vi "APXPressureReaderEPICS.vi"() -> ()   [LabVIEW 2015]
uses:
  <vilib>/Instr/_visa.llb/VISA Configure Serial Port (Instr).vi
  <userlib>/caLab/Private/Get_PV-1D.vi
  <userlib>/caLab/Private/Put_DBL-1D_PV-1D.vi
panel:
  out "VISA resource name out":refnum<visa-resource-name>
  out "APX:Gas":dbl format="%_3f"
  out "APX:Gas2":dbl format="%_3f"
  out "read buffer Main":string
  out "COM MAXGAUGE":refnum<visa-resource-name>
  out "Status":bool
  out "APX:SP_F":bool
  out "APX:SP_E":bool
  out "APX_SP_D":bool
  out "APX:SP_C":bool
  out "APX:SP_B":bool
  out "APX:SP_A":bool
  out "Cycle":i32
  out "Error out":errorcluster
  out "APX:SEN6_VAL":dbl format="%.6f"
  out "APX:SEN5_VAL":dbl format="%#_3e"
  out "APX:SEN4_VAL":dbl format="%#_4g"
  out "APX:SEN3_VAL":dbl format="%#_3g"
  out "APX:SEN2_VAL":dbl format="%#_3g"
  out "APX:SEN1_VAL":dbl format="%.5g"
  out "APX:SEN6_OFF":bool
  out "APX:SEN6_ON":bool
  out "APX:SEN5_OFF":bool
  out "APX:SEN5_ON":bool
  out "APX:SEN4_OFF":bool
  out "APX:SEN4_ON":bool
  out "APX:SEN3_OFF":bool
  out "APX:SEN3_ON":bool
  out "APX:SEN2_OFF":bool
  out "APX:SEN2_ON":bool
  out "APX:SEN1_OFF":bool
  out "APX:SEN1_ON":bool
  in  "STOP":bool
  # "APX:SP_SES100"
  # "APX:HPC100"
  # "APX:HPC"
  # "APX:PREP"
  # "APX:AP1"
  # "APX:AP2"
  # "APX:HPC01"
  # "APX:GAS"
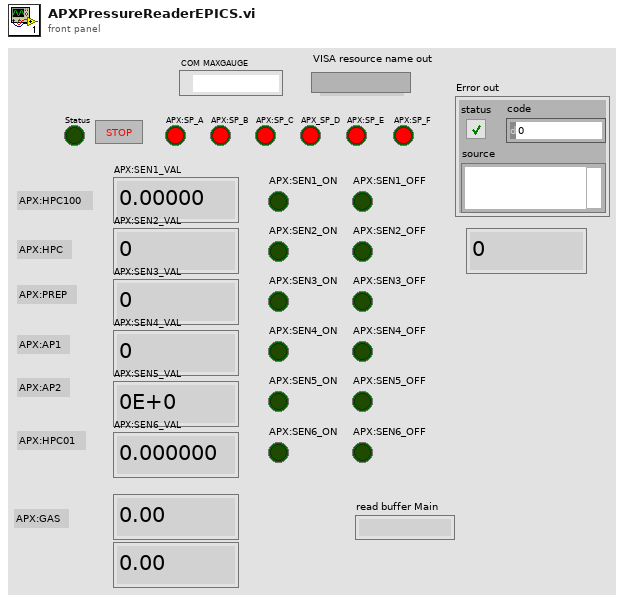
[diagram p1: front panel]
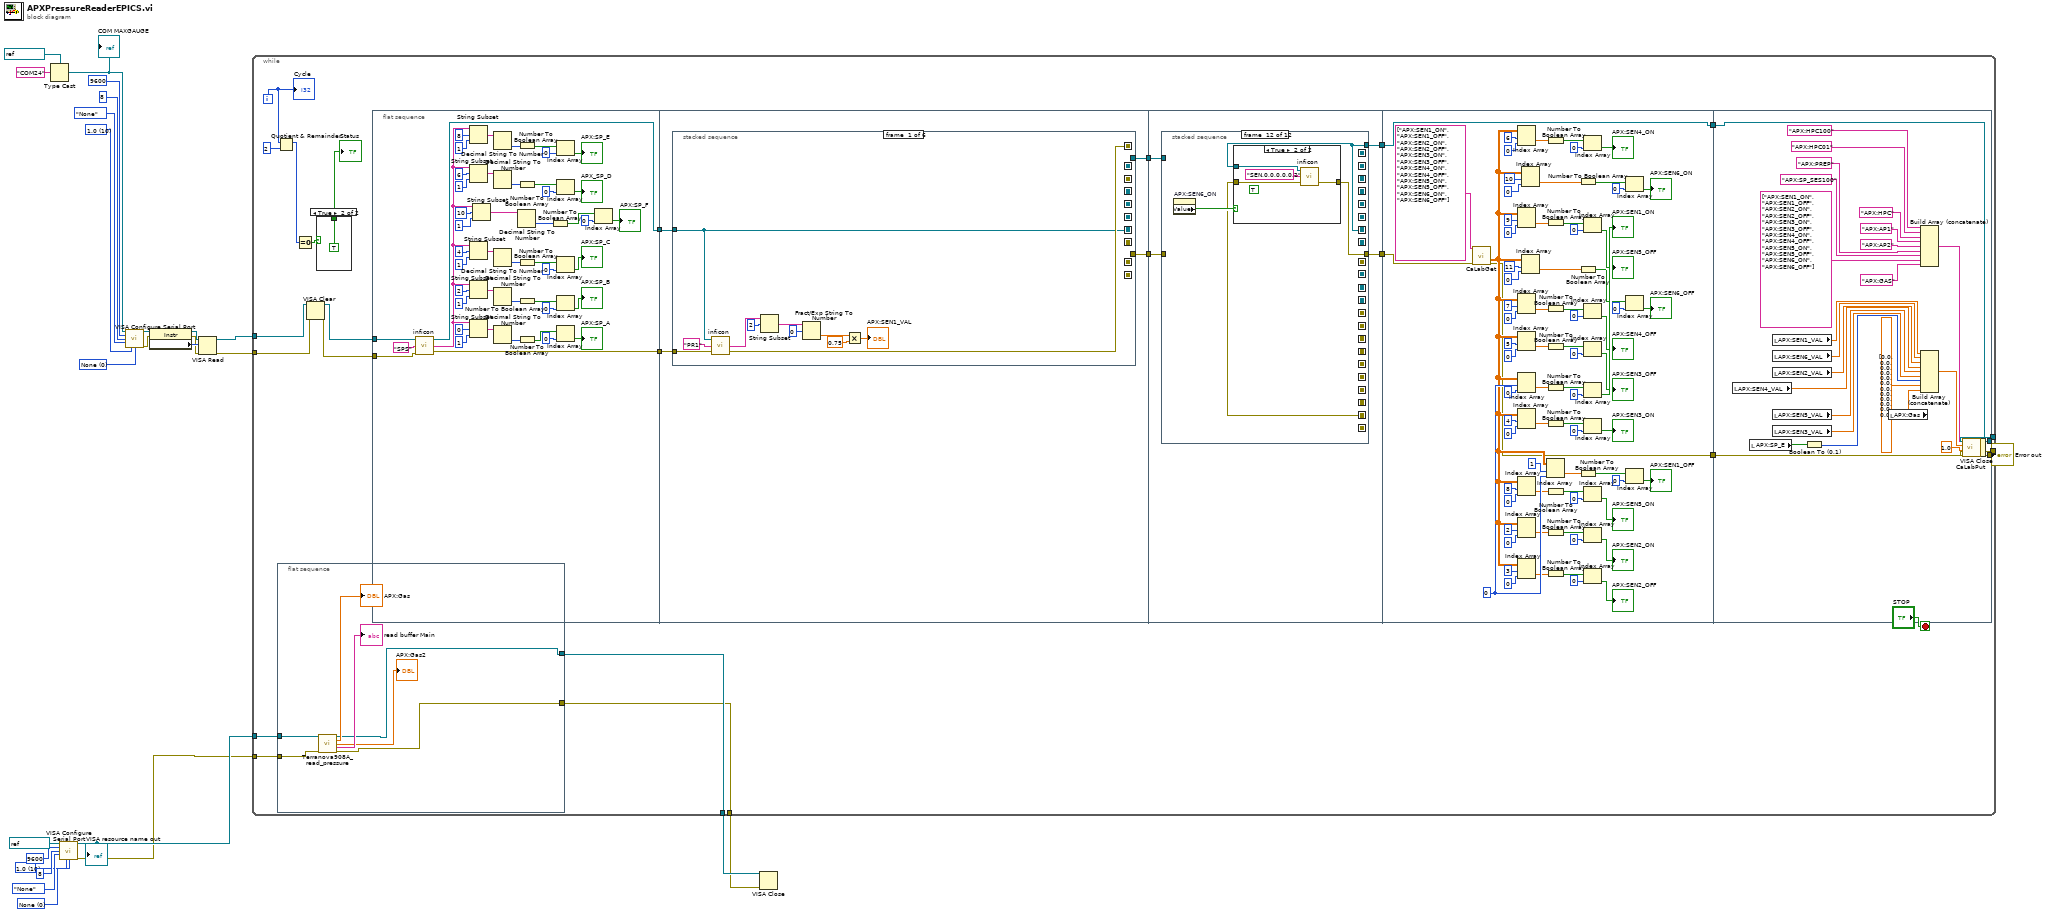
[diagram p0: block diagram]
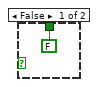
[diagram p2: hidden frame]
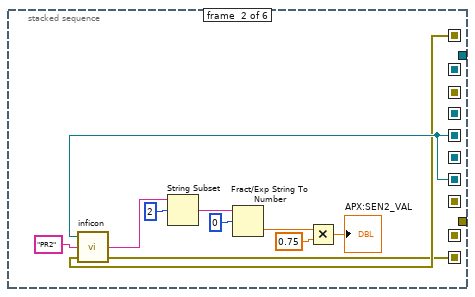
[diagram p3: hidden frame]
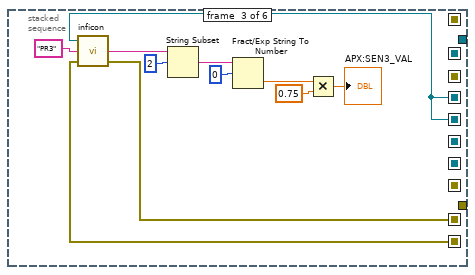
[diagram p4: hidden frame]
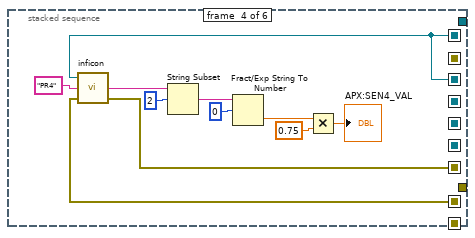
[diagram p5: hidden frame]
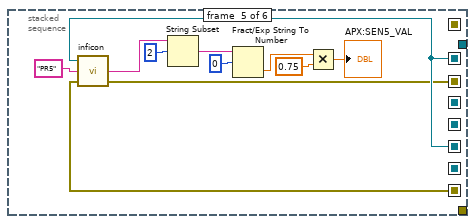
[diagram p6: hidden frame]
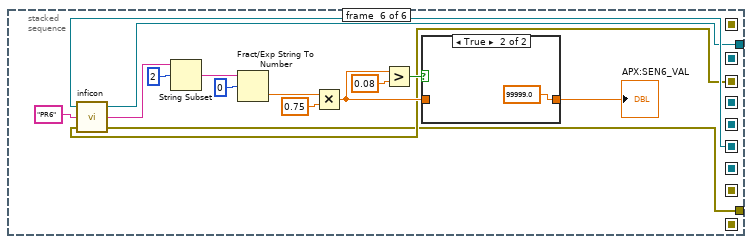
[diagram p7: hidden frame]
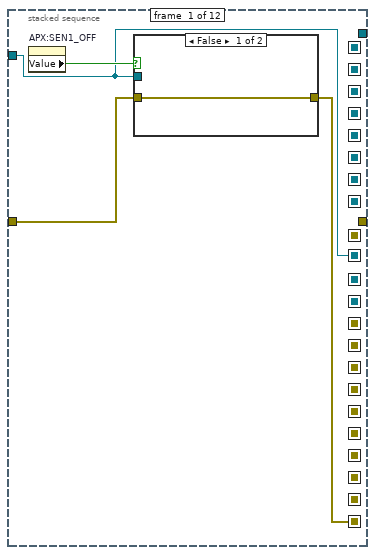
[diagram p9: hidden frame]
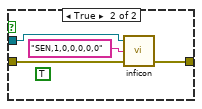
[diagram p10: hidden frame]
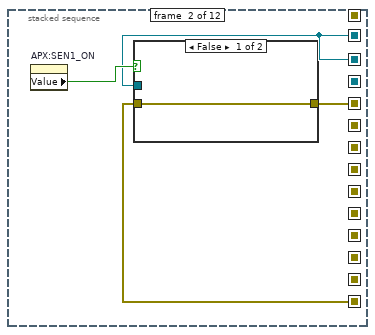
[diagram p11: hidden frame]
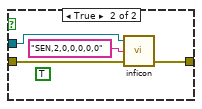
[diagram p12: hidden frame]
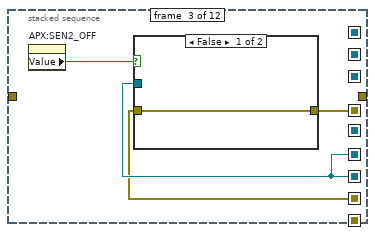
[diagram p13: hidden frame]
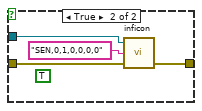
[diagram p14: hidden frame]
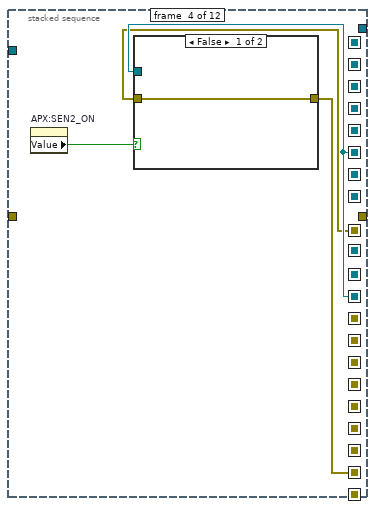
[diagram p15: hidden frame]
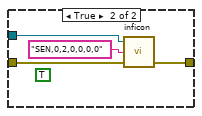
[diagram p16: hidden frame]
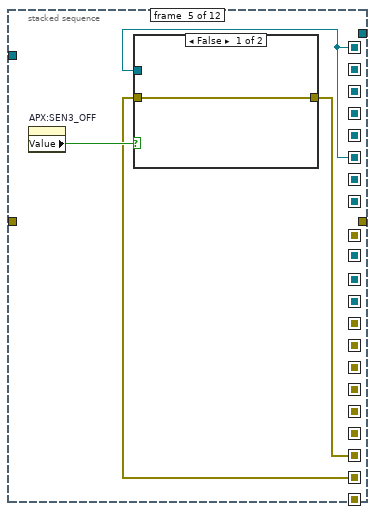
[diagram p17: hidden frame]
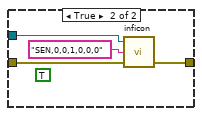
[diagram p18: hidden frame]
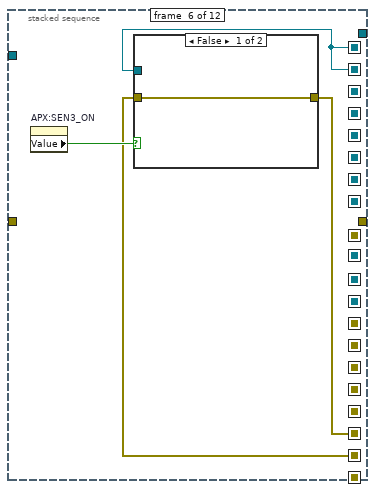
[diagram p19: hidden frame]
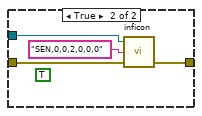
[diagram p20: hidden frame]
diagram:
  w5 = u16 10 items=["1.0"=10, "1.5"=15, "2.0"=20] ("stop bits (10: 1 bit)")
  w6 = u16 0 items=["None", "XON/XOFF", "RTS/CTS", "XON/XOFF & RTS/CTS", "DTR/DSR", "XON/XOFF & DTR/DSR"] ("flow control (0:none)")
  w24 = u16 10 items=["1.0"=10, "1.5"=15, "2.0"=20] ("stop bits (10: 1 bit)")
  w25 = u16 0 items=["None", "XON/XOFF", "RTS/CTS", "XON/XOFF & RTS/CTS", "DTR/DSR", "XON/XOFF & DTR/DSR"] ("flow control (0:none)")
  n1 = Type Cast(type=refnum<visa-resource-name> "COM24" ("VISA resource name"), x="COM24") -> (*(type *) &x=w22:refnum<visa-resource-name>)
  "COM MAXGAUGE" <- w22
  n2 = call-poly "VISA Configure Serial Port"("VISA resource name"=refnum<visa-resource-name> "COM10", "baud rate (9600)"=u32 9600, "data bits (8)"=u16 8, "parity (0:none)"=enum16{"None", "Odd", "Even", "Mark", "Space"}."None", "stop bits (10: 1 bit)"=w5, "flow control (0:none)"=w6) -> ("VISA resource name out"=w2:refnum<visa-resource-name>, "error out"=w1:errorcluster)  [unwired: 8 in]
  "VISA resource name out" <- w2
  n3 = call-poly "VISA Configure Serial Port"("VISA resource name"=w22, "baud rate (9600)"=u32 9600, "data bits (8)"=u16 8, "parity (0:none)"=enum16{"None", "Odd", "Even", "Mark", "Space"}."None", "stop bits (10: 1 bit)"=w24, "flow control (0:none)"=w25) -> ("VISA resource name out"=w19:refnum<visa-resource-name>, "error out"=w11:errorcluster)  [unwired: 8 in]
  n4 = property class="Instr"(reference=w19, error in=w11) -> (reference out=w20:refnum<visa-resource-name>, error out=w12:errorcluster, "Serial Settings:Number of Bytes at Serial Port"=w17:u32)
  n5 = VISA Read(VISA resource name=w20, byte count=w17, error in (no error)=w12) -> (VISA resource name out=w18:refnum<visa-resource-name>, error out=w13:errorcluster)  [unwired: 2 out]
  n6 = while {
    tunnel: [w46] -> w15
    tunnel: w18 -> [w41]
    tunnel: [w49] -> w16
    tunnel: w13 -> [w39]
    tunnel: [w32] -> w4
    tunnel: [w31] -> w3
    tunnel: w2 -> [w30]
    tunnel: w1 -> [w29]
    i -> [w35]
    stop <- "STOP" stop-if-true
    n7 = Quotient & Remainder(x=w35, y=2) -> (x-y*floor(x/y)=w36:i32)  [unwired: 1 out]
    n8 = flat-sequence {
      tunnel: w30 -> [w59]
      tunnel: [w57] -> w31
      tunnel: [w54] -> w32
      tunnel: w29 -> [w53]
      frame #0 {
        n9 = call "Terranova908A_read_pressure.vi"("VISA resource name"=w59, "error in (no error)"=w53) -> ("VISA resource name out"=w54:refnum<visa-resource-name>, "pressure"=→"APX:Gas":dbl, "pressure 2"=→"APX:Gas2":dbl, "read buffer"=→"read buffer Main":string, "error out"=w57:errorcluster)  [unwired: 9 in]
      }
    }
    n10 = Equal To 0?(x=w36) -> (x = 0?=w37:bool)
    n11 = VISA Clear(VISA resource name=w41, error in (no error)=w39) -> (VISA resource name out=w40:refnum<visa-resource-name>, error out=w38:errorcluster)
    n12 = case shown="True" w37 {
      tunnel: [FALSE ("Status") TRUE ("Status")] -> w33
      frame False {
      }
      frame True {
      }
    }
    "Status" <- w33
    n13 = flat-sequence {
      tunnel: w40 -> [w101]
      tunnel: [w100] -> w51
      tunnel: [w63] -> w45
      tunnel: w38 -> [w62]
      tunnel: w51 -> [w112]
      tunnel: [w111] -> w50
      tunnel: w45 -> [w113]
      tunnel: [w110] -> w44
      tunnel: w50 -> [w189]
      tunnel: w44 -> [w188]
      tunnel: [w187] -> w43
      tunnel: [w186] -> w42
      tunnel: [w300] -> w48
      tunnel: [w299] -> w47
      tunnel: w43 -> [w298]
      tunnel: w42 -> [w299]
      tunnel: [w398] -> w49
      tunnel: w48 -> [w376]
      tunnel: w47 -> [w398]
      tunnel: [w377] -> w46
      frame #0 {
        n14 = call "inficon.vi"("error out"=w62, "string to write"="SPS", "VISA resource name"=w101) -> ("error out 2"=w63:errorcluster, "read buffer 2"=w69:string, "VISA resource name 2"=w100:refnum<visa-resource-name>)
        n15 = String Subset(string=w69, offset (0)=8, length (rest)=1 ("length (rest)")) -> (substring=w103:string)
        n16 = String Subset(string=w69, offset (0)=6, length (rest)=1 ("length (rest)")) -> (substring=w88:string)
        n17 = String Subset(string=w69, offset (0)=4, length (rest)=1 ("length (rest)")) -> (substring=w94:string)
        n18 = String Subset(string=w69, offset (0)=2, length (rest)=1 ("length (rest)")) -> (substring=w82:string)
        n19 = String Subset(string=w69, offset (0)=0, length (rest)=1 ("length (rest)")) -> (substring=w76:string)
        n20 = String Subset(string=w69, offset (0)=10, length (rest)=1 ("length (rest)")) -> (substring=w70:string)
        n21 = Decimal String To Number(string=w103) -> (number=w104:i32)  [unwired: 2 in, 1 out]
        n22 = Decimal String To Number(string=w88) -> (number=w89:i32)  [unwired: 2 in, 1 out]
        n23 = Decimal String To Number(string=w94) -> (number=w95:i32)  [unwired: 2 in, 1 out]
        n24 = Decimal String To Number(string=w82) -> (number=w83:i32)  [unwired: 2 in, 1 out]
        n25 = Decimal String To Number(string=w76) -> (number=w77:i32)  [unwired: 2 in, 1 out]
        n26 = Decimal String To Number(string=w70) -> (number=w71:i32)  [unwired: 2 in, 1 out]
        n27 = Number To Boolean Array(number=w104) -> (Boolean array=w106:bool[])
        n28 = Number To Boolean Array(number=w89) -> (Boolean array=w91:bool[])
        n29 = Number To Boolean Array(number=w95) -> (Boolean array=w97:bool[])
        n30 = Number To Boolean Array(number=w83) -> (Boolean array=w85:bool[])
        n31 = Number To Boolean Array(number=w77) -> (Boolean array=w79:bool[])
        n32 = Number To Boolean Array(number=w71) -> (Boolean array=w73:bool[])
        n33 = Index Array(array=w106, index=0) -> (element=→"APX:SP_E":bool)
        n34 = Index Array(array=w91, index=0) -> (element=→"APX_SP_D":bool)
        n35 = Index Array(array=w97, index=0) -> (element=→"APX:SP_C":bool)
        n36 = Index Array(array=w85, index=0) -> (element=→"APX:SP_B":bool)
        n37 = Index Array(array=w79, index=0) -> (element=→"APX:SP_A":bool)
        n38 = Index Array(array=w73, index=0) -> (element=→"APX:SP_F":bool)
      }
      frame #1 {
        n39 = stacked-sequence {
          seq-local: [w114 _ _ _ _ _] -> [_ w135 _ _ _ _]
          seq-local: [w116 _ _ _ _ _] -> [_ w126 _ _ _ _]
          seq-local: [_ w135 _ _ _ _] -> [_ _ w146 _ _ _]
          seq-local: [_ w125 _ _ _ _] -> [_ _ w137 _ _ _]
          seq-local: [_ _ w146 _ _ _] -> [_ _ _ w157 _ _]
          seq-local: [_ _ w136 _ _ _] -> [_ _ _ w148 _ _]
          seq-local: [_ _ _ w157 _ _] -> [_ _ _ _ w168 _]
          seq-local: [_ _ _ w147 _ _] -> [_ _ _ _ w158 _]
          seq-local: [_ _ _ _ w168 _] -> [_ _ _ _ _ w183]
          seq-local: [_ _ _ _ w159 _] -> [_ _ _ _ _ w171]
          tunnel: w112 -> [w114 _ _ _ _ _]
          tunnel: w113 -> [w115 _ _ _ _ _]
          tunnel: [_ _ _ _ _ w170] -> w110
          tunnel: [_ _ _ _ _ w169] -> w111
          frame #0 {
            n40 = call "inficon.vi"("error out"=w115, "string to write"="PR1", "VISA resource name"=w114) -> ("error out 2"=w116:errorcluster, "read buffer 2"=w122:string)  [unwired: 1 out]
            n41 = String Subset(string=w122, offset (0)=2) -> (substring=w121:string)  [unwired: 1 in]
            n42 = Fract/Exp String To Number(string=w121, offset=0) -> (number=w117:dbl)  [unwired: 3 out]
            n43 = Multiply(x=w117, y=0.75) -> (x*y=→"APX:SEN1_VAL":dbl)
          }
          frame #1 {
            n44 = call "inficon.vi"("error out"=w126, "string to write"="PR2", "VISA resource name"=w135) -> ("error out 2"=w125:errorcluster, "read buffer 2"=w132:string)  [unwired: 1 out]
            n45 = String Subset(string=w132, offset (0)=2) -> (substring=w131:string)  [unwired: 1 in]
            n46 = Fract/Exp String To Number(string=w131, offset=0) -> (number=w127:dbl)  [unwired: 2 in, 1 out]
            n47 = Multiply(x=w127, y=0.75) -> (x*y=→"APX:SEN2_VAL":dbl)
          }
          frame #2 {
            n48 = call "inficon.vi"("error out"=w137, "string to write"="PR3", "VISA resource name"=w146) -> ("error out 2"=w136:errorcluster, "read buffer 2"=w143:string)  [unwired: 1 out]
            n49 = String Subset(string=w143, offset (0)=2) -> (substring=w141:string)  [unwired: 1 in]
            n50 = Fract/Exp String To Number(string=w141, offset=0 ("offset (0)")) -> (number=w138:dbl)  [unwired: 3 out]
            n51 = Multiply(x=w138, y=0.75) -> (x*y=→"APX:SEN3_VAL":dbl)
          }
          frame #3 {
            n52 = call "inficon.vi"("error out"=w148, "string to write"="PR4", "VISA resource name"=w157) -> ("error out 2"=w147:errorcluster, "read buffer 2"=w154:string)  [unwired: 1 out]
            n53 = String Subset(string=w154, offset (0)=2) -> (substring=w152:string)  [unwired: 1 in]
            n54 = Fract/Exp String To Number(string=w152, offset=0 ("offset (0)")) -> (number=w149:dbl)  [unwired: 3 out]
            n55 = Multiply(x=w149, y=0.75) -> (x*y=→"APX:SEN4_VAL":dbl)
          }
          frame #4 {
            n56 = call "inficon.vi"("error out"=w158, "string to write"="PR5", "VISA resource name"=w168) -> ("error out 2"=w159:errorcluster, "read buffer 2"=w165:string)  [unwired: 1 out]
            n57 = String Subset(string=w165, offset (0)=2) -> (substring=w163:string)  [unwired: 1 in]
            n58 = Fract/Exp String To Number(string=w163, offset=0 ("offset (0)")) -> (number=w160:dbl)  [unwired: 3 out]
            n59 = Multiply(x=w160, y=0.75) -> (x*y=→"APX:SEN5_VAL":dbl)
          }
          frame #5 {
            n60 = call "inficon.vi"("error out"=w171, "string to write"="PR6", "VISA resource name"=w183) -> ("error out 2"=w170:errorcluster, "read buffer 2"=w180:string, "VISA resource name 2"=w169:refnum<visa-resource-name>)
            n61 = String Subset(string=w180, offset (0)=2) -> (substring=w178:string)  [unwired: 1 in]
            n62 = Fract/Exp String To Number(string=w178, offset=0 ("offset (0)")) -> (number=w172:dbl)  [unwired: 3 out]
            n63 = Multiply(x=w172, y=0.75) -> (x*y=w175:dbl)
            n64 = Greater?(x=w175, y=0.08) -> (0:w177:bool)
            n65 = case shown="True" w177 {
              tunnel: w175 -> [w184 _]
              tunnel: [w184 99999.0 ("y")] -> w176
              frame False {
              }
              frame True {
              }
            }
            "APX:SEN6_VAL" <- w176
          }
        }
      }
      frame #2 {
        n66 = stacked-sequence {
          seq-local: [w192 _ _ _ _ _ _ _ _ _ _ _] -> [_ w201 _ _ _ _ _ _ _ _ _ _]
          seq-local: [w190 _ _ _ _ _ _ _ _ _ _ _] -> [_ w200 _ _ _ _ _ _ _ _ _ _]
          seq-local: [_ w201 _ _ _ _ _ _ _ _ _ _] -> [_ _ w210 _ _ _ _ _ _ _ _ _]
          seq-local: [_ w199 _ _ _ _ _ _ _ _ _ _] -> [_ _ w209 _ _ _ _ _ _ _ _ _]
          seq-local: [_ _ w210 _ _ _ _ _ _ _ _ _] -> [_ _ _ w219 _ _ _ _ _ _ _ _]
          seq-local: [_ _ w208 _ _ _ _ _ _ _ _ _] -> [_ _ _ w218 _ _ _ _ _ _ _ _]
          seq-local: [_ _ _ w219 _ _ _ _ _ _ _ _] -> [_ _ _ _ w228 _ _ _ _ _ _ _]
          seq-local: [_ _ _ w217 _ _ _ _ _ _ _ _] -> [_ _ _ _ w227 _ _ _ _ _ _ _]
          seq-local: [_ _ _ _ w228 _ _ _ _ _ _ _] -> [_ _ _ _ _ w237 _ _ _ _ _ _]
          seq-local: [_ _ _ _ w226 _ _ _ _ _ _ _] -> [_ _ _ _ _ w236 _ _ _ _ _ _]
          seq-local: [_ _ _ _ _ w237 _ _ _ _ _ _] -> [_ _ _ _ _ _ w246 _ _ _ _ _]
          seq-local: [_ _ _ _ _ w235 _ _ _ _ _ _] -> [_ _ _ _ _ _ w245 _ _ _ _ _]
          seq-local: [_ _ _ _ _ _ w246 _ _ _ _ _] -> [_ _ _ _ _ _ _ w255 _ _ _ _]
          seq-local: [_ _ _ _ _ _ w244 _ _ _ _ _] -> [_ _ _ _ _ _ _ w254 _ _ _ _]
          seq-local: [_ _ _ _ _ _ _ w255 _ _ _ _] -> [_ _ _ _ _ _ _ _ w264 _ _ _]
          seq-local: [_ _ _ _ _ _ _ w253 _ _ _ _] -> [_ _ _ _ _ _ _ _ w263 _ _ _]
          seq-local: [_ _ _ _ _ _ _ _ w264 _ _ _] -> [_ _ _ _ _ _ _ _ _ w273 _ _]
          seq-local: [_ _ _ _ _ _ _ _ w262 _ _ _] -> [_ _ _ _ _ _ _ _ _ w272 _ _]
          seq-local: [_ _ _ _ _ _ _ _ _ w273 _ _] -> [_ _ _ _ _ _ _ _ _ _ w282 _]
          seq-local: [_ _ _ _ _ _ _ _ _ w271 _ _] -> [_ _ _ _ _ _ _ _ _ _ w281 _]
          seq-local: [_ _ _ _ _ _ _ _ _ _ w282 _] -> [_ _ _ _ _ _ _ _ _ _ _ w289]
          seq-local: [_ _ _ _ _ _ _ _ _ _ w280 _] -> [_ _ _ _ _ _ _ _ _ _ _ w291]
          tunnel: w189 -> [w192 _ _ _ _ _ _ _ _ _ _ _]
          tunnel: w188 -> [w191 _ _ _ _ _ _ _ _ _ _ _]
          tunnel: [_ _ _ _ _ _ _ _ _ _ _ w290] -> w187
          tunnel: [_ _ _ _ _ _ _ _ _ _ _ w289] -> w186
          frame #0 {
            n67 = property on="APX:SEN1_OFF" class="Bool (strict)"() -> ("Value"=w193:bool)  [unwired: 2 in, 2 out]
            n68 = case shown="False" w193 {
              tunnel: w192 -> [_ w197]
              tunnel: w191 -> [w194 w196]
              tunnel: [w194 w195] -> w190
              frame False {
              }
              frame True {
                (unwired) TRUE ("Write/Read")
                n69 = call "inficon.vi"("error out"=w196, "string to write"="SEN,1,0,0,0,0,0" ("Command"), "VISA resource name"=w197) -> ("error out 2"=w195:errorcluster)  [unwired: 2 out]
              }
            }
          }
          frame #1 {
            n70 = property on="APX:SEN1_ON" class="Bool (strict)"() -> ("Value"=w202:bool)  [unwired: 2 in, 2 out]
            n71 = case shown="False" w202 {
              tunnel: w201 -> [_ w206]
              tunnel: w200 -> [w203 w205]
              tunnel: [w203 w204] -> w199
              frame False {
              }
              frame True {
                (unwired) TRUE ("Write/Read")
                n72 = call "inficon.vi"("error out"=w205, "string to write"="SEN,2,0,0,0,0,0" ("Command"), "VISA resource name"=w206) -> ("error out 2"=w204:errorcluster)  [unwired: 2 out]
              }
            }
          }
          frame #2 {
            n73 = property on="APX:SEN2_OFF" class="Bool (strict)"() -> ("Value"=w211:bool)  [unwired: 2 in, 2 out]
            n74 = case shown="False" w211 {
              tunnel: w210 -> [_ w215]
              tunnel: w209 -> [w212 w214]
              tunnel: [w212 w213] -> w208
              frame False {
              }
              frame True {
                (unwired) TRUE ("Write/Read")
                n75 = call "inficon.vi"("error out"=w214, "string to write"="SEN,0,1,0,0,0,0" ("Command"), "VISA resource name"=w215) -> ("error out 2"=w213:errorcluster)  [unwired: 2 out]
              }
            }
          }
          frame #3 {
            n76 = property on="APX:SEN2_ON" class="Bool (strict)"() -> ("Value"=w220:bool)  [unwired: 2 in, 2 out]
            n77 = case shown="False" w220 {
              tunnel: w219 -> [_ w224]
              tunnel: w218 -> [w221 w223]
              tunnel: [w221 w222] -> w217
              frame False {
              }
              frame True {
                (unwired) TRUE ("Write/Read")
                n78 = call "inficon.vi"("error out"=w223, "string to write"="SEN,0,2,0,0,0,0" ("Command"), "VISA resource name"=w224) -> ("error out 2"=w222:errorcluster)  [unwired: 2 out]
              }
            }
          }
          frame #4 {
            n79 = property on="APX:SEN3_OFF" class="Bool (strict)"() -> ("Value"=w229:bool)  [unwired: 2 in, 2 out]
            n80 = case shown="False" w229 {
              tunnel: w228 -> [_ w233]
              tunnel: w227 -> [w230 w232]
              tunnel: [w230 w231] -> w226
              frame False {
              }
              frame True {
                (unwired) TRUE ("Write/Read")
                n81 = call "inficon.vi"("error out"=w232, "string to write"="SEN,0,0,1,0,0,0" ("Command"), "VISA resource name"=w233) -> ("error out 2"=w231:errorcluster)  [unwired: 2 out]
              }
            }
          }
          frame #5 {
            n82 = property on="APX:SEN3_ON" class="Bool (strict)"() -> ("Value"=w238:bool)  [unwired: 2 in, 2 out]
            n83 = case shown="False" w238 {
              tunnel: w237 -> [_ w242]
              tunnel: w236 -> [w239 w241]
              tunnel: [w239 w240] -> w235
              frame False {
              }
              frame True {
                (unwired) TRUE ("Write/Read")
                n84 = call "inficon.vi"("error out"=w241, "string to write"="SEN,0,0,2,0,0,0" ("Command"), "VISA resource name"=w242) -> ("error out 2"=w240:errorcluster)  [unwired: 2 out]
              }
            }
          }
          frame #6 {
            n85 = property on="APX:SEN4_OFF" class="Bool (strict)"() -> ("Value"=w247:bool)  [unwired: 2 in, 2 out]
            n86 = case shown="True" w247 {
              tunnel: w246 -> [_ w251]
              tunnel: w245 -> [w248 w250]
              tunnel: [w248 w249] -> w244
              frame False {
              }
              frame True {
                (unwired) TRUE ("Write/Read")
                n87 = call "inficon.vi"("error out"=w250, "string to write"="SEN,0,0,0,1,0,0" ("Command"), "VISA resource name"=w251) -> ("error out 2"=w249:errorcluster)  [unwired: 2 out]
              }
            }
          }
          frame #7 {
            n88 = property on="APX:SEN4_ON" class="Bool (strict)"() -> ("Value"=w256:bool)  [unwired: 2 in, 2 out]
            n89 = case shown="False" w256 {
              tunnel: w255 -> [_ w260]
              tunnel: w254 -> [w257 w259]
              tunnel: [w257 w258] -> w253
              frame False {
              }
              frame True {
                (unwired) TRUE ("Write/Read")
                n90 = call "inficon.vi"("error out"=w259, "string to write"="SEN,0,0,0,2,0,0" ("Command"), "VISA resource name"=w260) -> ("error out 2"=w258:errorcluster)  [unwired: 2 out]
              }
            }
          }
          frame #8 {
            n91 = property on="APX:SEN5_OFF" class="Bool (strict)"() -> ("Value"=w265:bool)  [unwired: 2 in, 2 out]
            n92 = case shown="False" w265 {
              tunnel: w264 -> [_ w269]
              tunnel: w263 -> [w266 w268]
              tunnel: [w266 w267] -> w262
              frame False {
              }
              frame True {
                (unwired) TRUE ("Write/Read")
                n93 = call "inficon.vi"("error out"=w268, "string to write"="SEN,0,0,0,0,1,0" ("Command"), "VISA resource name"=w269) -> ("error out 2"=w267:errorcluster)  [unwired: 2 out]
              }
            }
          }
          frame #9 {
            n94 = property on="APX:SEN5_ON" class="Bool (strict)"() -> ("Value"=w274:bool)  [unwired: 2 in, 2 out]
            n95 = case shown="False" w274 {
              tunnel: w273 -> [_ w278]
              tunnel: w272 -> [w275 w277]
              tunnel: [w275 w276] -> w271
              frame False {
              }
              frame True {
                (unwired) TRUE ("Write/Read")
                n96 = call "inficon.vi"("error out"=w277, "string to write"="SEN,0,0,0,0,2,0" ("Command"), "VISA resource name"=w278) -> ("error out 2"=w276:errorcluster)  [unwired: 2 out]
              }
            }
          }
          frame #10 {
            n97 = property on="APX:SEN6_OFF" class="Bool (strict)"() -> ("Value"=w283:bool)  [unwired: 2 in, 2 out]
            n98 = case shown="False" w283 {
              tunnel: w282 -> [_ w287]
              tunnel: w281 -> [w284 w286]
              tunnel: [w284 w285] -> w280
              frame False {
              }
              frame True {
                (unwired) TRUE ("Write/Read")
                n99 = call "inficon.vi"("error out"=w286, "string to write"="SEN,0,0,0,0,0,1" ("Command"), "VISA resource name"=w287) -> ("error out 2"=w285:errorcluster)  [unwired: 2 out]
              }
            }
          }
          frame #11 {
            n100 = property on="APX:SEN6_ON" class="Bool (strict)"() -> ("Value"=w292:bool)  [unwired: 2 in, 2 out]
            n101 = case shown="True" w292 {
              tunnel: w289 -> [_ w296]
              tunnel: w291 -> [w293 w295]
              tunnel: [w293 w294] -> w290
              frame False {
              }
              frame True {
                (unwired) TRUE ("Write/Read")
                n102 = call "inficon.vi"("error out"=w295, "string to write"="SEN,0,0,0,0,0,2" ("Command"), "VISA resource name"=w296) -> ("error out 2"=w294:errorcluster)  [unwired: 2 out]
              }
            }
          }
        }
      }
      frame #3 {
        w363 = 0 ("index")
        n103 = call-poly "CaLabGet.vi"("PV Names"=string[] ["APX:SEN1_ON", "APX:SEN1_OFF", "APX:SEN2_ON", "APX:SEN2_OFF", "APX:SEN3_ON", "APX:SEN3_OFF", "APX:SEN4_ON", "APX:SEN4_OFF", "APX:SEN5_ON", "APX:SEN5_OFF", "APX:SEN6_ON", "APX:SEN6_OFF"], "Error in (no error)"=w298) -> ("Value Array (number)"=w322:dbl[][], "Error out"=w300:errorcluster)  [unwired: 7 in, 5 out]
        n104 = Index Array(array=w322, index (row)=6 ("disabled index (col)"), index (col)=0) -> (element=w311:dbl)
        n105 = Index Array(array=w322, index (row)=9 ("disabled index (col)"), index (col)=0) -> (element=w305:dbl)
        n106 = Index Array(array=w322, index (row)=7 ("disabled index (col)"), index (col)=0) -> (element=w309:dbl)
        n107 = Index Array(array=w322, index (row)=5 ("disabled index (col)"), index (col)=0) -> (element=w313:dbl)
        n108 = Index Array(array=w322, index (row)=w363, index (col)=0 ("disabled index (col)")) -> (element=w371:dbl)
        n109 = Index Array(array=w322, index (row)=4 ("disabled index (col)"), index (col)=0) -> (element=w315:dbl)
        n110 = Index Array(array=w322, index (row)=8 ("disabled index (col)"), index (col)=0) -> (element=w307:dbl)
        n111 = Index Array(array=w322, index (row)=2 ("disabled index (col)"), index (col)=0) -> (element=w319:dbl)
        n112 = Index Array(array=w322, index (row)=3 ("disabled index (col)"), index (col)=0) -> (element=w317:dbl)
        n113 = Index Array(array=w322, index (row)=10 ("disabled index (col)"), index (col)=0) -> (element=w303:dbl)
        n114 = Index Array(array=w322, index (row)=11 ("disabled index (col)"), index (col)=0) -> (element=w301:dbl)
        n115 = Index Array(array=w322, index (row)=1 ("disabled index (col)"), index (col)=w363) -> (element=w367:dbl)
        n116 = Number To Boolean Array(number=w311) -> (Boolean array=w345:bool[])
        n117 = Number To Boolean Array(number=w305) -> (Boolean array=w333:bool[])
        n118 = Number To Boolean Array(number=w309) -> (Boolean array=w341:bool[])
        n119 = Number To Boolean Array(number=w313) -> (Boolean array=w349:bool[])
        n120 = Number To Boolean Array(number=w371) -> (Boolean array=w370:bool[])
        n121 = Number To Boolean Array(number=w315) -> (Boolean array=w353:bool[])
        n122 = Number To Boolean Array(number=w307) -> (Boolean array=w337:bool[])
        n123 = Number To Boolean Array(number=w319) -> (Boolean array=w361:bool[])
        n124 = Number To Boolean Array(number=w317) -> (Boolean array=w357:bool[])
        n125 = Number To Boolean Array(number=w303) -> (Boolean array=w329:bool[])
        n126 = Number To Boolean Array(number=w301) -> (Boolean array=w325:bool[])
        n127 = Number To Boolean Array(number=w367) -> (Boolean array=w366:bool[])
        n128 = Index Array(array=w345, index=0) -> (element=→"APX:SEN4_ON":bool)
        n129 = Index Array(array=w333, index=0) -> (element=→"APX:SEN5_OFF":bool)
        n130 = Index Array(array=w341, index=0) -> (element=→"APX:SEN4_OFF":bool)
        n131 = Index Array(array=w349, index=0) -> (element=→"APX:SEN3_OFF":bool)
        n132 = Index Array(array=w370, index=0) -> (element=→"APX:SEN1_ON":bool)
        n133 = Index Array(array=w353, index=0) -> (element=→"APX:SEN3_ON":bool)
        n134 = Index Array(array=w337, index=0) -> (element=→"APX:SEN5_ON":bool)
        n135 = Index Array(array=w361, index=0) -> (element=→"APX:SEN2_ON":bool)
        n136 = Index Array(array=w357, index=0) -> (element=→"APX:SEN2_OFF":bool)
        n137 = Index Array(array=w329, index=0) -> (element=→"APX:SEN6_ON":bool)
        n138 = Index Array(array=w325, index=0) -> (element=→"APX:SEN6_OFF":bool)
        n139 = Index Array(array=w366, index=0) -> (element=→"APX:SEN1_OFF":bool)
      }
      frame #4 {
        n140 = local read "APX:SEN4_VAL"() -> (w395:dbl)
        n141 = local read "APX:SP_E"() -> (w396:bool)
        n142 = local read "APX:SEN1_VAL"() -> (w391:dbl)
        n143 = local read "APX:SEN6_VAL"() -> (w394:dbl)
        n144 = local read "APX:SEN2_VAL"() -> (w392:dbl)
        n145 = local read "APX:SEN5_VAL"() -> (w393:dbl)
        n146 = local read "APX:SEN3_VAL"() -> (w390:dbl)
        n147 = Boolean To (0,1)(Boolean=w396) -> (0, 1=w397:i16)
        n148 = local read "APX:Gas"() -> (w374:dbl)
        n149 = Build Array (concatenate)("APX:HPC100", "APX:HPC01", "APX:HPC", "APX:AP1", "APX:AP2", "APX:PREP", "APX:SP_SES100" ("element"), string[] ["APX:SEN1_ON", "APX:SEN1_OFF", "APX:SEN2_ON", "APX:SEN2_OFF", "APX:SEN3_ON", "APX:SEN3_OFF", "APX:SEN4_ON", "APX:SEN4_OFF", "APX:SEN5_ON", "APX:SEN5_OFF", "APX:SEN6_ON", "APX:SEN6_OFF"], "APX:GAS") -> (w379:string[])
        n150 = Build Array (concatenate)(w391, w394, w392, w395, w393, w390, w397, dbl[] [0.0, 0.0, 0.0, 0.0, 0.0, 0.0, 0.0, 0.0, 0.0, 0.0, 0.0, 0.0], w374) -> (w378:dbl[])
        n151 = call-poly <userlib>:"CaLabPut.vi"("Error in (no error)"=w376, "Timeout (3)"=1.0, "Values"=w378, "PV Names"=w379) -> ("Error out"=w377:errorcluster)  [unwired: 4 in, 3 out]
      }
    }
    "Cycle" <- w35
  }
  n152 = VISA Close(VISA resource name=w4, error in (no error)=w3) -> ()  [unwired: 1 out]
  n153 = VISA Close(VISA resource name=w16, error in (no error)=w15) -> (error out=→"Error out":errorcluster)
